vi "TRF to TSP Plot.vi"(8 "Transport Graph Properties":T1={"Transport Line Size"=0, "Transport Line Color"=16774656} {"Transport Line Size" items=["Extra Small", "Small", "Medium", "Large", "Extra Large"]}, 11 "Transfer File":path) -> (1 "Transport":cluster{ext[], ext[]}[](graph), 2 "Transport File":path, 3 "Transfer Folder":path)   [LabVIEW 2011]
uses:
  <vilib>/Utility/file.llb/Read From Spreadsheet File (string).vi
panel:
  out "Transport Name":string
  out "No Transport File":path
  out "Transport Folder":path
  in  "default (0 dbl)":ext format="%.2e"
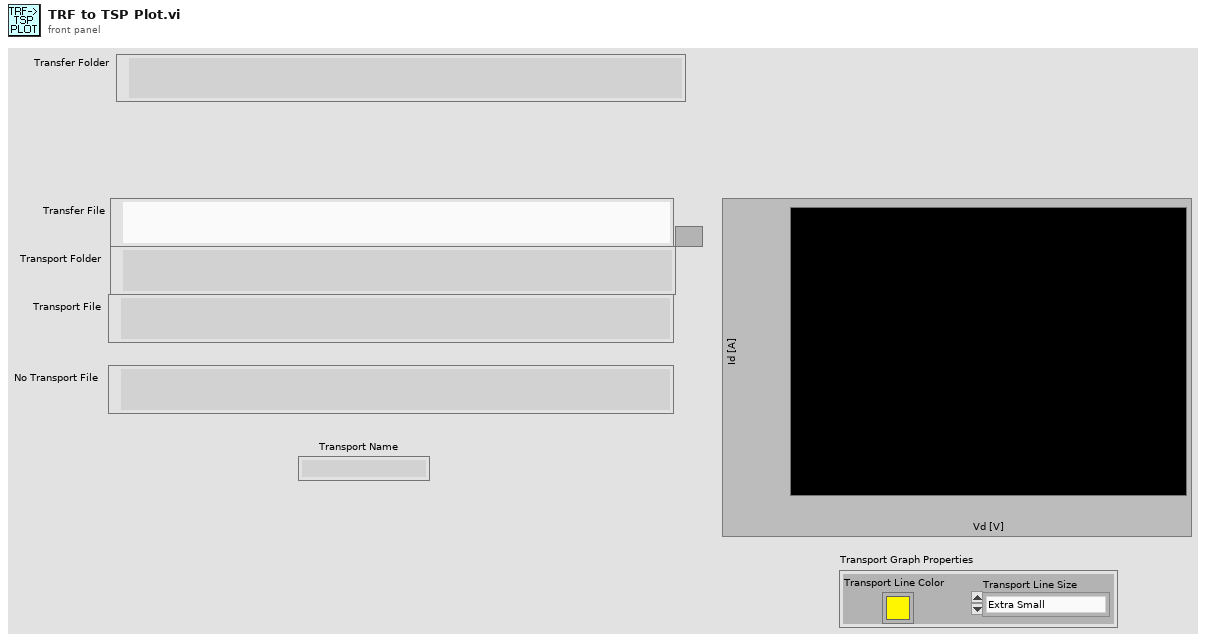
[diagram p1: front panel]
types:
  T1 = cluster{"Transport Line Size":u16, "Transport Line Color":u32}
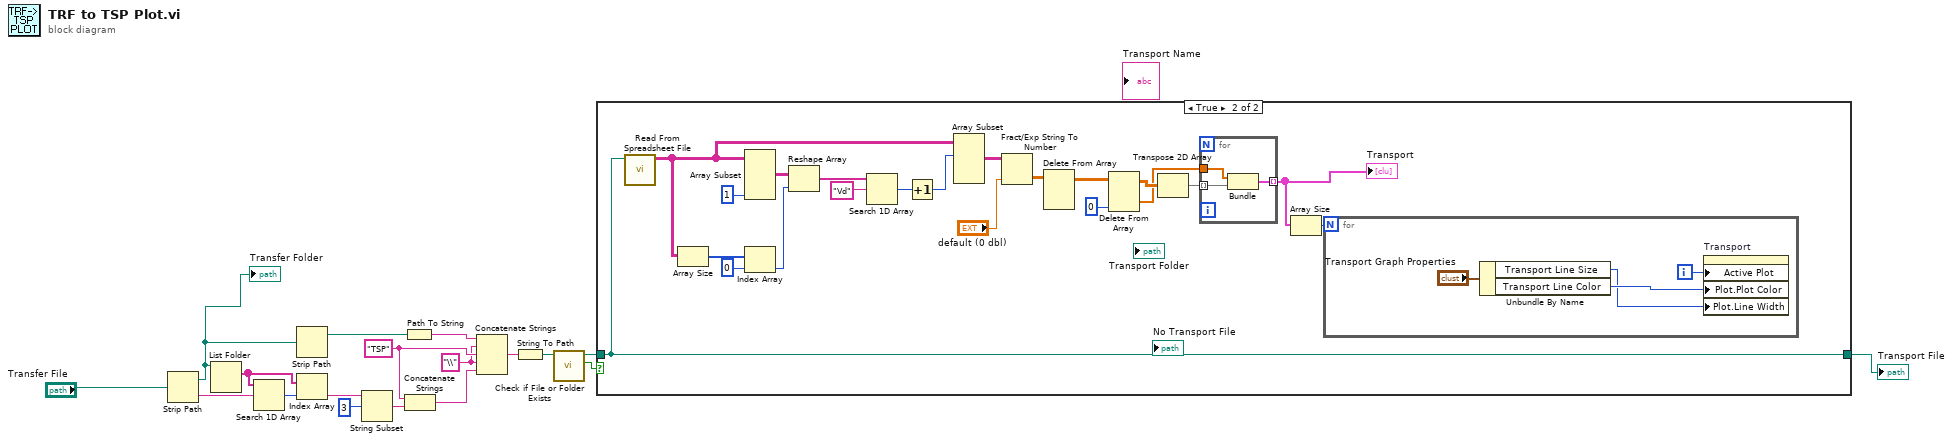
[diagram p0: block diagram]
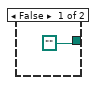
[diagram p2: hidden frame]
diagram:
  w13 = "\\"
  w14 = "TSP"
  n1 = Strip Path(path="Transfer File") -> (stripped path=w2:path, name=w15:string)
  "Transfer Folder" <- w2
  n2 = List Folder(path=w2) -> (filenames=w17:string[])  [unwired: 3 in, 3 out]
  n3 = Search 1D Array(1D array=w17, element=w15) -> (index of element=w16:i32)  [unwired: 1 in]
  n4 = Strip Path(path=w2) -> (stripped path=w9:path)  [unwired: 1 out]
  n5 = Index Array(array=w17, index=w16) -> (element=w18:string)
  n6 = String Subset(string=w18, offset (0)=3) -> (substring=w8:string)  [unwired: 1 in]
  n7 = Path To String(path=w9) -> (string=w12:string)
  n8 = Concatenate Strings(w14, w8) -> (w10:string)
  n9 = Concatenate Strings(w12, w13, w14, w13, w10) -> (w11:string)
  n10 = String To Path(string=w11) -> (path=w6:path)
  n11 = call <vilib>:"Check if File or Folder Exists.vi"("path"=w6) -> ("file or folder exists?"=w5:bool, "dup path"=w4:path)  [unwired: 8 in, 1 out]
  n12 = case shown="True" w5 {
    tunnel: w4 -> [_ w20]
    tunnel: [path "" w20] -> w1
    frame False {
    }
    frame True {
      n13 = call-poly <vilib>:"Read From Spreadsheet File.vi"("file path (dialog if empty)"=w20) -> ("all rows"=w34:string[][])  [unwired: 6 in, 4 out]
      n14 = Array Size(array=w34) -> (size(s)=w40:i32[])
      n15 = Array Subset(array=w34, length (col)=1) -> (w36:string[][])  [unwired: 3 in]
      n16 = Index Array(array=w40, index=0) -> (element=w29:i32)
      n17 = Reshape Array(w36, w29) -> (w35:string[])
      n18 = Search 1D Array(1D array=w35, element="Vd") -> (index of element=w33:i32)  [unwired: 1 in]
      n19 = Increment(x=w33) -> (x+1=w32:i32)
      n20 = Array Subset(array=w34, index (row)=w32) -> (w30:string[][])  [unwired: 3 in]
      n21 = Fract/Exp String To Number(string=w30, default (0 dbl)="default (0 dbl)") -> (number=w23:ext[][])  [unwired: 2 in, 1 out]
      n22 = Delete From Array(array=w23) -> (array with subset deleted=w22:ext[][])  [unwired: 3 in, 1 out]
      n23 = Delete From Array(array=w22, index (col)=0 ("Deaktivierter Index (Spalte)")) -> (deleted portion=w26:ext[], array with subset deleted=w27:ext[][])  [unwired: 2 in]
      n24 = Transpose 2D Array(2D array=w27) -> (transposed array=w28:ext[][])
      n25 = for {
        tunnel: w26 -> [w46]
        tunnel: w28 -> [w47] mode=indexing
        tunnel: [w45] -> w21 mode=indexing
        n26 = Bundle(w46, w47) -> (w45:cluster{ext[], ext[]})  [unwired: 1 in]
      }
      "Transport" <- w21
      n27 = Array Size(array=w21) -> (size(s)=w24:i32)
      n28 = for {
        N: w24 -> [_]
        i -> [w44]
        n29 = Unbundle By Name("Transport Graph Properties") -> ("Transport Line Size"=w41:u16, "Transport Line Color"=w42:u32)
        n30 = property on="Transport" class="XYGraph (strict)"("Active Plot"=w44, "Plot.Plot Color"=w42, "Plot.Line Width"=w41) -> ()  [unwired: 2 in, 2 out]
      }
    }
  }
  "Transport File" <- w1
